vi "valve_pressures.vi"() -> ()   [LabVIEW 2016]
panel:
  out "Scroll Pump Pressure (mbar)":dbl format="%.2f"
  out "Chamber Pressure (mbar)":dbl format="%.2f"
  in  "stop":bool
  # "Turbo Pump"
  # "Scroll (Roughing) Pump"
  # "Pump"
  # "Back\nPressure\nReadout"
  # "Gate"
  # "Roughing"
  # "Chamber\nPressure\nReadout"
  # "Chamber"
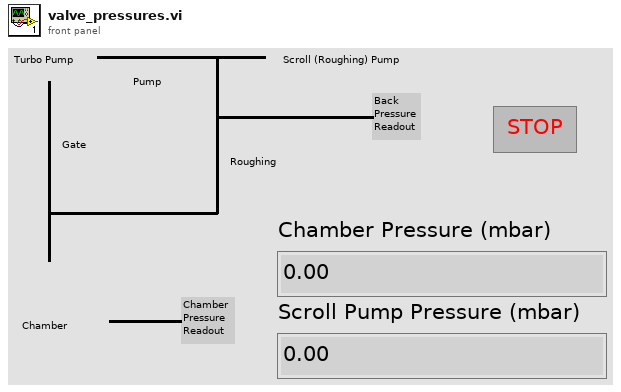
[diagram p1: front panel]
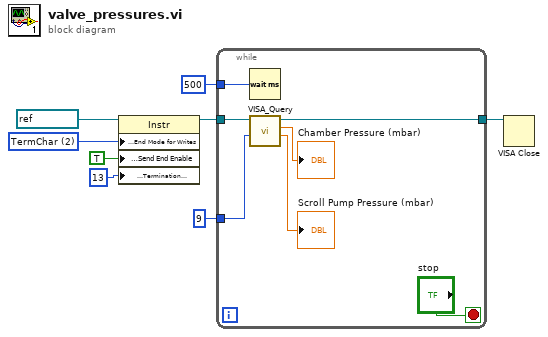
[diagram p0: block diagram]
diagram:
  w7 = u16 2 items=["None", "Last Bit", "TermChar", "Break"] ("Serial Settings:End Mode for Writes")
  n1 = property class="Instr"(reference=refnum<visa-resource-name> "COM8" ("VISA resource name"), "Serial Settings:End Mode for Writes"=w7, "Message Based Settings:Send End Enable"=TRUE, "Message Based Settings:Termination Character"=u8 13) -> (reference out=w4:refnum<visa-resource-name>)  [unwired: 1 in, 1 out]
  n2 = while {
    tunnel: w4 -> [w14]
    tunnel: u32 9 -> [w13]
    tunnel: [w12] -> w2
    tunnel: u32 500 ("milliseconds to wait") -> [w11]
    stop <- "stop" stop-if-true
    n3 = Wait (ms)(milliseconds to wait=w11) -> ()  [unwired: 1 out]
    n4 = call "VISA_Query.vi"("Byte Count"=w13, "VISA Refnum in"=w14) -> ("Scroll Pump Pressure (mbar)"=→"Scroll Pump Pressure (mbar)":dbl, "Chamber Pressure (mbar)"=→"Chamber Pressure (mbar)":dbl, "VISA Refnum out"=w12:refnum<visa-resource-name>)  [unwired: 7 in]
  }
  n5 = VISA Close(VISA resource name=w2) -> ()  [unwired: 1 in, 1 out]
